vi "sg Set AM.vi"(7 "shape":u32(ring) items=["sgShapeSine", "sgShapeTriangle", "sgShapeSquare", "sgShapeRamp"], 8 "error in (no error)":errorcluster, 9 "depth":dbl, 10 "frequency":dbl, 11 "device":i32) -> (0 "error out":errorcluster, 3 "function return":u32(ring))   [LabVIEW 2014, in "VSG25A.lvlib"]
doc: "SG_API sgStatus sgSetAM(int device, double frequency, double depth, sgShape shape);"
uses:
  VSG25A.lvlib
  sg_api.dll
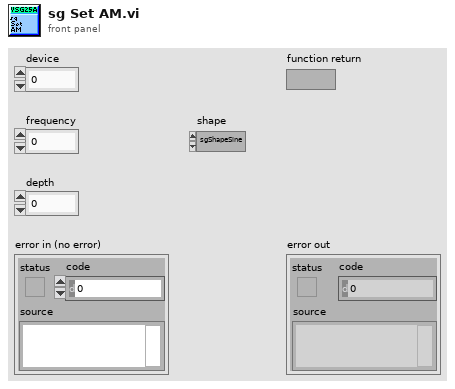
[diagram p1: front panel]
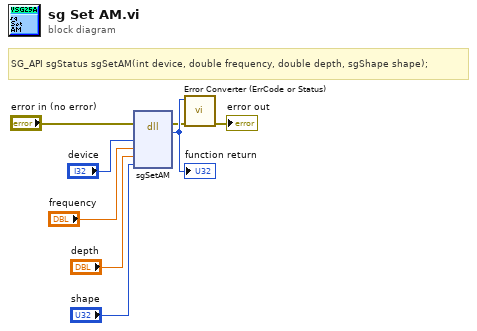
[diagram p0: block diagram]
diagram:
  # "SG_API sgStatus sgSetAM(int device, double frequency, double depth, sgShape shape);"
  n1 = dll-call lib="C:/Users/M_LAPTOP/Desktop/Labview/practice/VSG25A/sg_lib/sg_api.*" fn="sgSetAM"(error in="error in (no error)", "device"="device", "frequency"="frequency", "depth"="depth", "shape"="shape") -> (error out=w2:errorcluster, w8:u32)  [unwired: 6 in, 1 out]
  "function return" <- w8
  n2 = call "Error Converter (ErrCode or Status).vi"("error in (no error)"=w2, "error code"=w8) -> ("error out"=→"error out":errorcluster)  [unwired: 9 in]
